vi "test_Multiple Local Array Format Channel Command-Response Messages using Trigger with Padding and Protection.vi"(8 "error in (no error)":errorcluster, 11 "TestCase in":refnum<class "Instrument Addon Common System Tests.lvclass">) -> (0 "error out":errorcluster, 3 "TestCase out":refnum<class "Instrument Addon Common System Tests.lvclass">)   [LabVIEW 2019, in "Instrument Addon Common System Tests.lvclass"]
uses:
  Instrument Addon Common System Tests.lvclass
  <vilib>/addons/_JKI Toolkits/VI Tester/TestCase.llb/TestCase.lvclass
  <vilib>/NI VeriStand/Execution/Workspace/NI_VS Workspace ExecutionAPI.lvlib
  <vilib>/NI VeriStand/Execution/Workspace/NI VeriStand - Get Multiple Channel Values.vi
  <vilib>/NI VeriStand/Execution/Workspace/NI VeriStand - Set Multiple Channel Values.vi
  C:/Users/nitest/Desktop/Git 2019/niveristand-custom-device-testing-tools/VeriStandTestCase/VeriStandTestCase.lvclass
  C:/Program Files (x86)/National Instruments/LabVIEW 2019/vi.lib/addons/_JKI Toolkits/VI Tester/TestCase.llb/TestCase.lvclass
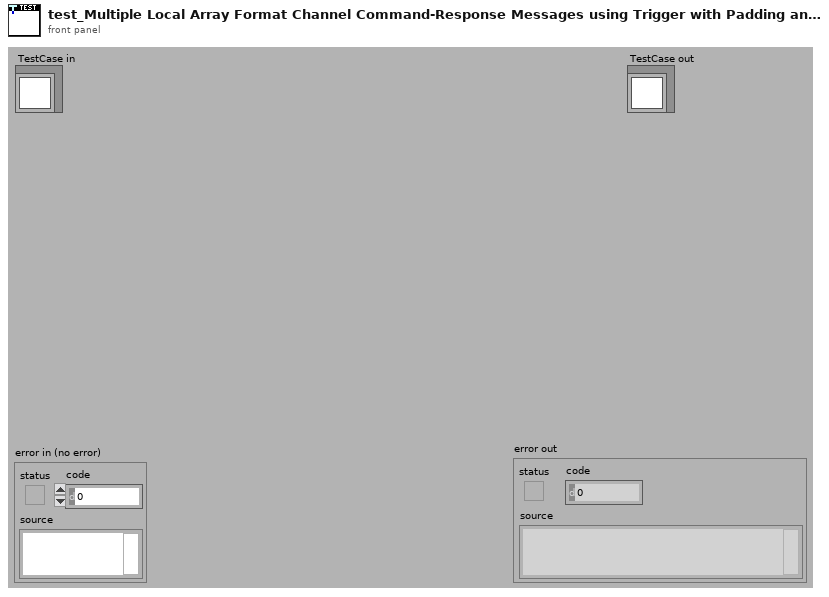
[diagram p1: front panel]
types:
  T1 = typedef "NI_VS Workspace ExecutionAPI.lvlib/WorkspaceAPI.ctl" = refnum<k24>
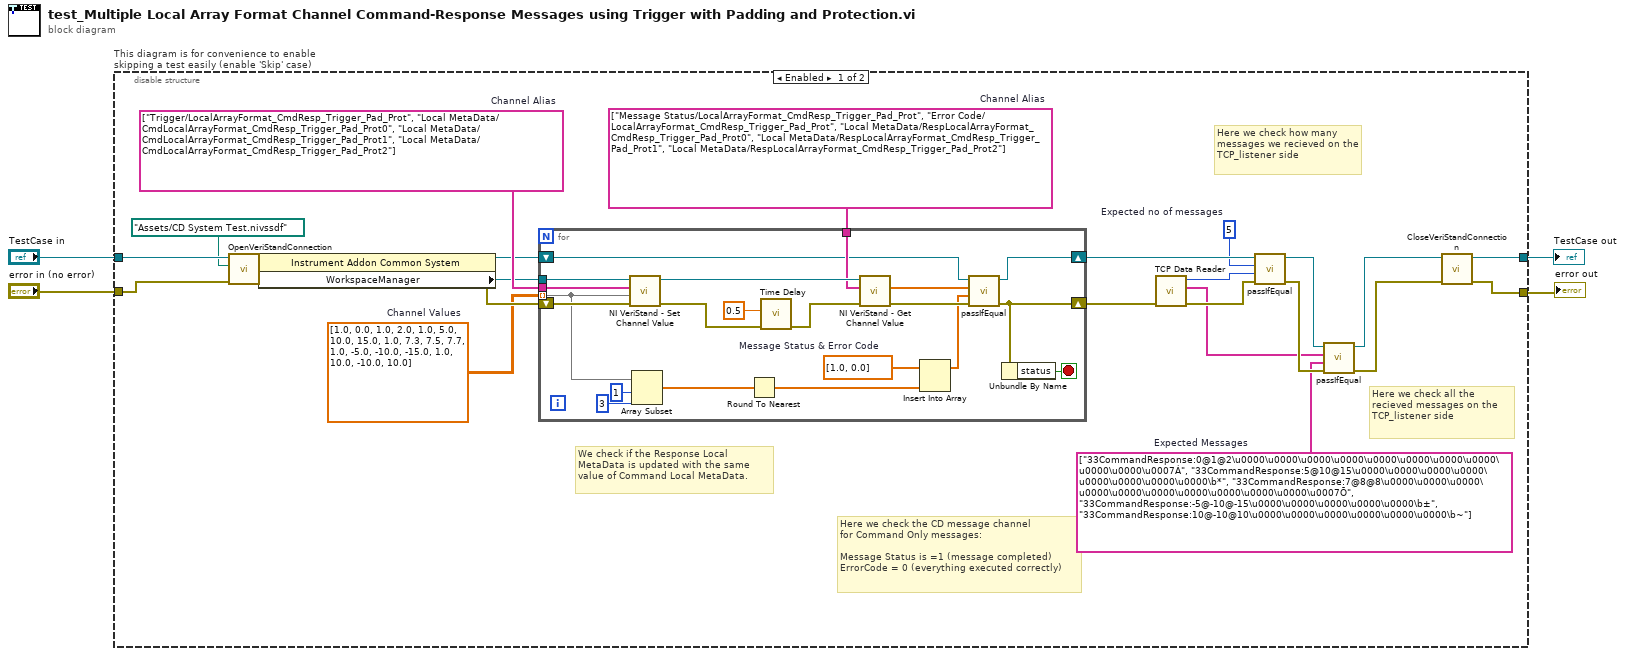
[diagram p0: block diagram]
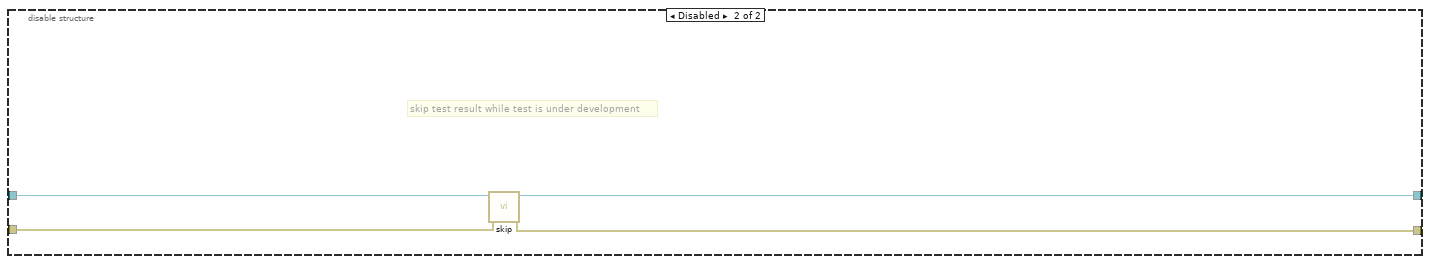
[diagram p2: hidden frame]
diagram:
  n1 = disable-structure "This diagram is for convenience to enable skipping a test easily (enable 'Skip' case)" shown="Enabled" {
    disable-tunnel: "TestCase in" -> [w26 w53]
    disable-tunnel: [w27 w51] -> w1
    disable-tunnel: [w28 w52] -> w3
    disable-tunnel: "error in (no error)" -> [w24 w50]
    frame Enabled {
      w5 = string[] ["33CommandResponse:0@1@2\u0000\u0000\u0000\u0000\u0000\u0000\u0000\u0000\u0000\u0000\u0007Á", "33CommandResponse:5@10@15\u0000\u0000\u0000\u0000\u0000\u0000\u0000\u0000\b*", "33CommandResponse:7@8@8\u0000\u0000\u0000\u0000\u0000\u0000\u0000\u0000\u0000\u0000\u0007Õ", "33CommandResponse:-5@-10@-15\u0000\u0000\u0000\u0000\u0000\b±", "33CommandResponse:10@-10@10\u0000\u0000\u0000\u0000\u0000\u0000\b~"]  # Expected Messages
      w8 = 5  # Expected no of messages
      w17 = string[] ["Message Status/LocalArrayFormat_CmdResp_Trigger_Pad_Prot", "Error Code/LocalArrayFormat_CmdResp_Trigger_Pad_Prot", "Local MetaData/RespLocalArrayFormat_CmdResp_Trigger_Pad_Prot0", "Local MetaData/RespLocalArrayFormat_CmdResp_Trigger_Pad_Prot1", "Local MetaData/RespLocalArrayFormat_CmdResp_Trigger_Pad_Prot2"]  # Channel Alias
      w19 = dbl[][] [[1.0, 0.0, 1.0, 2.0], [1.0, 5.0, 10.0, 15.0], [1.0, 7.3, 7.5, 7.7], [1.0, -5.0, -10.0, -15.0], [1.0, 10.0, -10.0, 10.0]]  # Channel Values
      w20 = string[] ["Trigger/LocalArrayFormat_CmdResp_Trigger_Pad_Prot", "Local MetaData/CmdLocalArrayFormat_CmdResp_Trigger_Pad_Prot0", "Local MetaData/CmdLocalArrayFormat_CmdResp_Trigger_Pad_Prot1", "Local MetaData/CmdLocalArrayFormat_CmdResp_Trigger_Pad_Prot2"]  # Channel Alias
      # "We check if the Response Local MetaData is updated with the same value of Command Local MetaData."
      # "Here we check how many messages we recieved on the TCP_listener side"
      # "Here we check all the recieved messages on the TCP_listener side"
      # "Here we check the CD message channel\nfor Command Only messages:\n\nMessage Status is =1 (message completed)\nErrorCode = 0 (everything executed correctly)"
      n2 = call-dynamic "OpenVeriStandConnection.vi"("error in (no error)"=w24, "System Definition File"=path "Assets/CD System Test.nivssdf", "VeriStand Test Case in"=w26) -> ("error out"=w23:errorcluster, "VeriStand Test Case out"=w25:refnum<class "Instrument Addon Common System Tests.lvclass">)  [unwired: 6 in, 1 out]
      n3 = property class="Instrument Addon Common System "(reference=w25, error in=w23) -> (reference out=w18:refnum<class "Instrument Addon Common System Tests.lvclass">, error out=w21:errorcluster, "WorkspaceManager"=w16:T1)
      n4 = for {
        tunnel: w16 -> [w49]
        tunnel: w20 -> [w47]
        tunnel: w19 -> [w34] mode=indexing
        shift-right: [w36] -> w7
        shift-left: w21 -> [w48]
        tunnel: w17 -> [w45]
        shift-right: [w40] -> w15
        shift-left: w18 -> [w41]
        stop <- w35 stop-if-true
        w37 = dbl[] [1.0, 0.0]  # Message Status & Error Code
        n5 = call-poly <vilib>:"NI VeriStand - Set Channel Value.vi"("error in (no error)"=w48, "Values"=w34, "Channels"=w47, "WorkspaceManager in"=w49) -> ("error out"=w43:errorcluster, "WorkspaceManager out"=w46:T1)  [unwired: 6 in]
        n6 = Array Subset(array=w34, index=1, length=3 ("index")) -> (w31:dbl[])
        n7 = Round To Nearest(number=w31) -> (nearest integer value=w29:dbl[])
        n8 = call "Time Delay"("error in (no error)"=w43, "Delay Time (s)"=0.5) -> ("error out"=w42:errorcluster)  [unwired: 9 in]
        n9 = call-poly <vilib>:"NI VeriStand - Get Channel Value.vi"("error in (no error)"=w42, "Channels"=w45, "WorkspaceManager in"=w46) -> ("error out"=w39:errorcluster, "Values"=w38:dbl[])  [unwired: 6 in, 1 out]
        n10 = Insert Into Array(array=w37, new element=w29) -> (w33:dbl[])  [unwired: 1 in]
        n11 = call-dynamic "passIfEqual.vi"("error in (no error)"=w39, "y"=w33, "x"=w38, "TestCase in"=w41) -> ("error out"=w36:errorcluster, "TestCase out"=w40:refnum<class "Instrument Addon Common System Tests.lvclass">)  [unwired: 6 in]
        n12 = Unbundle By Name(w36) -> ("status"=w35:bool)
      }
      n13 = call "TCP Data Reader.vi"("error in (no error)"=w7) -> ("error out"=w13:errorcluster, "Recieved Messages"=w6:string[], "No of messages"=w9:i32)  [unwired: 8 in]
      n14 = call-dynamic "passIfEqual.vi"("error in (no error)"=w13, "y"=w9, "x"=w8, "TestCase in"=w15) -> ("error out"=w11:errorcluster, "TestCase out"=w14:refnum<class "Instrument Addon Common System Tests.lvclass">)  [unwired: 6 in]
      n15 = call-dynamic "passIfEqual.vi"("error in (no error)"=w11, "y"=w5, "x"=w6, "TestCase in"=w14) -> ("error out"=w10:errorcluster, "TestCase out"=w12:refnum<class "Instrument Addon Common System Tests.lvclass">)  [unwired: 6 in]
      n16 = call-dynamic "CloseVeriStandConnection.vi"("error in (no error)"=w10, "VeriStand Test Case in"=w12) -> ("error out"=w28:errorcluster, "VeriStand Test Case out"=w27:refnum<class "Instrument Addon Common System Tests.lvclass">)  [unwired: 8 in]
    }
    frame Disabled {
      # "skip test result while test is under development"
      n17 = call <vilib>:"skip.vi"("error in (no error)"=w50, "TestCase in"=w53) -> ("error out"=w52:errorcluster, "TestCase out"=w51:refnum<class "Instrument Addon Common System Tests.lvclass">)  [unwired: 8 in]
    }
  }
  "error out" <- w3
  "TestCase out" <- w1
